vi "cwlaserSelectorEnable.vi"(1 "wavelength":dbl) -> ()   [LabVIEW 2017]
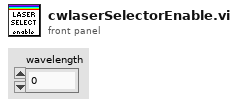
[diagram p1: front panel]
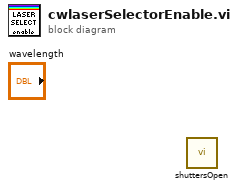
[diagram p0: block diagram]
diagram:
  n1 = call "shuttersOpen.vi"() -> ()  [unwired: 12 in]
